vi "Integrate Pulse.vi"(7 "Refnum Cluster in":T1, 8 "error in (no error)":errorcluster, 9 "Short Gate in":i32, 10 "Long Gate in":i32, 11 "DigitiserActor in":refnum<class "DigitiserActor.lvclass">) -> (0 "error out":errorcluster, 3 "DigitiserActor out":refnum<class "DigitiserActor.lvclass">)   [LabVIEW 2019, in "DigitiserActor.lvlib" / "DigitiserActor.lvclass"]
uses:
  DigitiserActor.lvclass
  DigitiserActor.lvclass/DigitiserActor.ctl
  <vilib>/Analysis/baseanly.llb/Mean (DBL).vi
  <vilib>/Analysis/NI_AALBase.lvlib
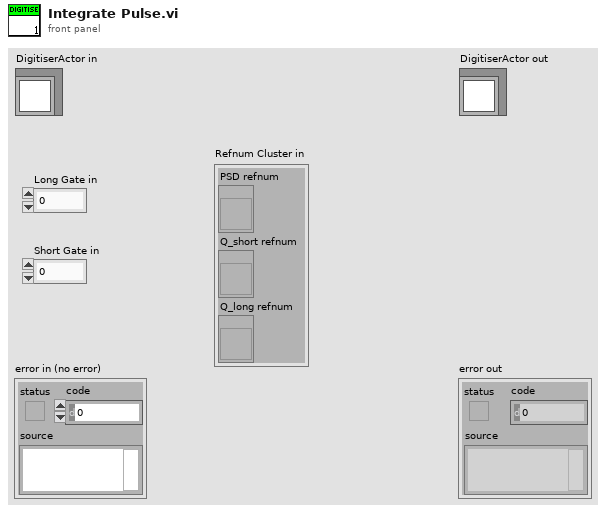
[diagram p1: front panel]
types:
  T1 = cluster{"PSD refnum":refnum<vi>, "Q_short refnum":refnum<vi>, "Q_long refnum":refnum<vi>}
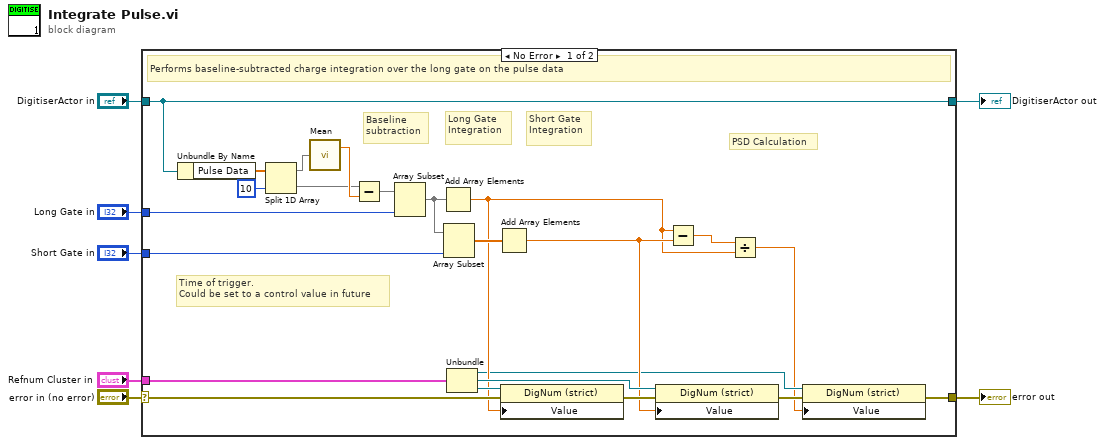
[diagram p0: block diagram]
diagram:
  n1 = case shown="No Error" "error in (no error)" {
    selector: "error in (no error)" -> [w22 w32]
    tunnel: [w10 w32] -> w6
    tunnel: [w30 w31] -> w4
    tunnel: "DigitiserActor in" -> [w30 w31]
    tunnel: "Long Gate in" -> [w24 _]
    tunnel: "Short Gate in" -> [w20 _]
    tunnel: "Refnum Cluster in" -> [w18 _]
    frame No Error {
      # "Time of trigger.\nCould be set to a control value in future"
      # "PSD Calculation"
      # "Short Gate Integration"
      # "Long Gate Integration"
      # "Baseline subtraction"
      # "Performs baseline-subtracted charge integration over the long gate on the pulse data"
      n2 = Unbundle By Name(w30) -> ("Pulse Data"=w29:dbl[])
      n3 = Split 1D Array(array=w29, index=10) -> (first subarray=w27:dbl[], second subarray=w25:dbl[])
      n4 = call-poly <vilib>:"Mean.vi"("X"=w27) -> ("mean"=w26:dbl)  [unwired: 1 out]
      n5 = Subtract(x=w25, y=w26) -> (x-y=w23:dbl[])
      n6 = Array Subset(array=w23, length=w24) -> (w21:dbl[])  [unwired: 1 in]
      n7 = Add Array Elements(numeric array=w21) -> (sum=w12:dbl)
      n8 = Array Subset(array=w21, length=w20) -> (w19:dbl[])  [unwired: 1 in]
      n9 = Unbundle(w18) -> ("PSD refnum"=w9:refnum<vi>, "Q_short refnum"=w16:refnum<vi>, "Q_long refnum"=w17:refnum<vi>)
      n10 = Add Array Elements(numeric array=w19) -> (sum=w14:dbl)
      n11 = property class="DigNum (strict)"(reference=w17, error in=w22, "Value"=w12) -> (error out=w15:errorcluster)  [unwired: 1 out]
      n12 = property class="DigNum (strict)"(reference=w16, error in=w15, "Value"=w14) -> (error out=w11:errorcluster)  [unwired: 1 out]
      n13 = Subtract(x=w12, y=w14) -> (x-y=w13:dbl)
      n14 = Divide(x=w13, y=w12) -> (x/y=w8:dbl)
      n15 = property class="DigNum (strict)"(reference=w9, error in=w11, "Value"=w8) -> (error out=w10:errorcluster)  [unwired: 1 out]
    }
    frame Error {
    }
  }
  "error out" <- w6
  "DigitiserActor out" <- w4
